vi "ChannelList_Attributes_GetPropertyNames.vi"(8 "error in (no error)":errorcluster, 10 "Channel ID":string, 11 "OXY_SCPI Reseource In":refnum<visa-resource-name>) -> (0 "error out":errorcluster, 1 "communication_data":T1, 2 "Property Names":string[](array[string]), 3 "OXY_SCPI Reseource Out":refnum<visa-resource-name>)   [LabVIEW 2020, in "OXYGEN_Datastream.lvlib"]
doc: "Queries the names (keys) of properties (config-items) of a given channel."
uses:
  OXYGEN_Datastream.lvlib
  TypeDefs/Cluster_RawCommData.ctl
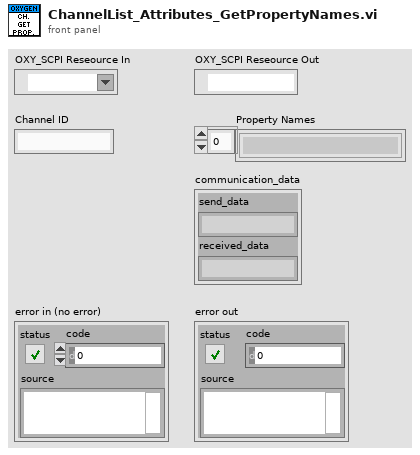
[diagram p1: front panel]
types:
  T1 = typedef "OXYGEN_Datastream.lvlib/Cluster_RawCommData.ctl" = cluster{"send_data":string, "received_data":string}
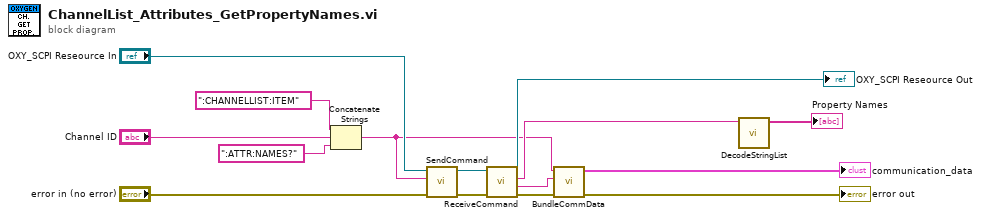
[diagram p0: block diagram]
diagram:
  n1 = Concatenate Strings(":CHANNELLIST:ITEM", "Channel ID", ":ATTR:NAMES?") -> (w1:string)
  n2 = call "SendCommand.vi"("error in (no error)"="error in (no error)", "String to Send"=w1, "OXY_SCPI Reseource In"="OXY_SCPI Reseource In") -> ("error out"=w14:errorcluster, "OXY_SCPI Reseource Out"=w13:refnum<visa-resource-name>)  [unwired: 7 in]
  n3 = call "ReceiveCommand.vi"("error in (no error)"=w14, "OXY_SCPI Reseource In"=w13) -> ("error out"=w9:errorcluster, "received Data with Header"=w7:string, "received Data"=w6:string, "OXY_SCPI Reseource Out"=→"OXY_SCPI Reseource Out":refnum<visa-resource-name>)  [unwired: 6 in]
  n4 = call "BundleCommData.vi"("error in (no error)"=w9, "received_data"=w7, "send_data"=w1) -> ("error out"=→"error out":errorcluster, "communication_data"=→"communication_data":T1)  [unwired: 7 in]
  n5 = call "DecodeStringList.vi"("String List (\"<STR1>\",\"<STR2>\",...)"=w6) -> ("String as Array"=→"Property Names":string[])  [unwired: 9 in, 1 out]
